vi "Create Configuration List.vi"(8 "error in (no error)":errorcluster, 9 "Configuration List Name":string="MyMeasList", 10 "Configuration List Type (0: Measure)":u16(ring) items=["Measure", "Source"], 11 "VISA resource name":refnum<visa-resource-name>) -> (0 "error out":errorcluster, 3 "VISA resource name out":refnum<visa-resource-name>)   [LabVIEW 2021, in "Keithley 2450.lvlib"]
doc: "Creates a Measure or Source Configuration List"
uses:
  <instrlib>/Keithley 2450/Keithley 2450.lvlib
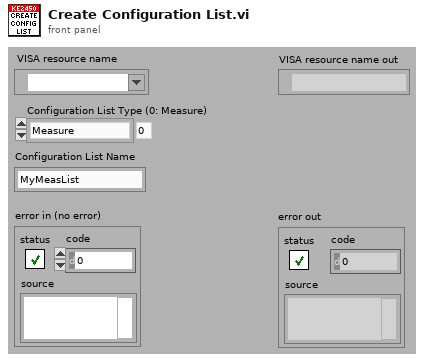
[diagram p1: front panel]
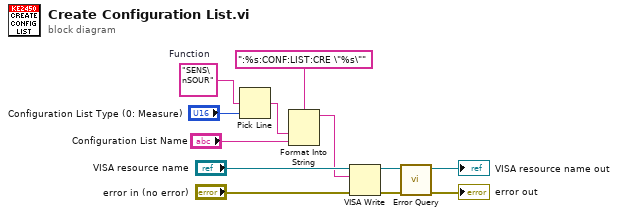
[diagram p0: block diagram]
diagram:
  w8 = "SENS\nSOUR"  # Function
  n1 = Pick Line(multi-line string=w8, line index="Configuration List Type (0: Measure)") -> (output string=w2:string)  [unwired: 1 out]
  n2 = Format Into String(format string=":%s:CONF:LIST:CRE \"%s\"", w2, "Configuration List Name") -> (resulting string=w4:string)  [unwired: 2 in, 1 out]
  n3 = VISA Write(VISA resource name="VISA resource name", write buffer=w4, error in (no error)="error in (no error)") -> (VISA resource name out=w6:refnum<visa-resource-name>, error out=w5:errorcluster)  [unwired: 1 out]
  n4 = call <instrlib>:"Error Query.vi"("error in (no error)"=w5, "VISA resource name"=w6) -> ("error out"=→"error out":errorcluster, "VISA resource name out"=→"VISA resource name out":refnum<visa-resource-name>)  [unwired: 8 out]
